vi "ATF-Storage NS Connect.vi"(8 "error in (no error)":errorcluster, 11 "Storage Ip Address":string) -> (0 "error out":errorcluster, 2 "writer endpoint":refnum<k21>, 3 "reader endpoint":refnum<k21>)   [LabVIEW 2022 SP3]
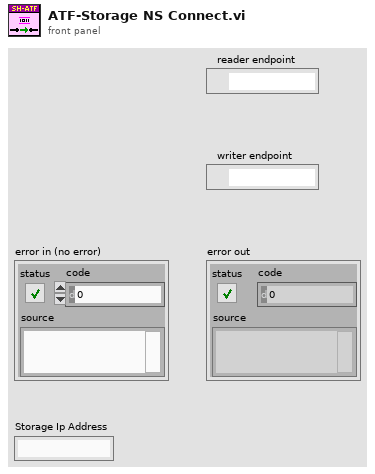
[diagram p1: front panel]
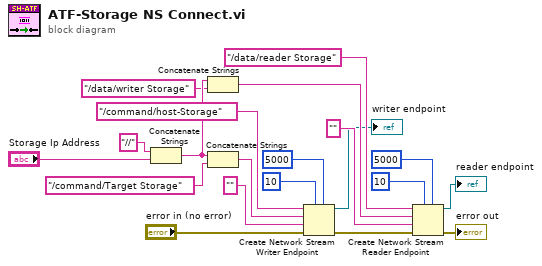
[diagram p0: block diagram]
diagram:
  n1 = Concatenate Strings("//" ("reader url"), "Storage Ip Address") -> (w16:string)
  n2 = Concatenate Strings(w16, "/data/writer Storage" ("reader url")) -> (w11:string)
  n3 = Concatenate Strings(w16, "/command/Target Storage" ("reader url")) -> (w12:string)
  n4 = Create Network Stream Writer Endpoint(5:5000 ("timeout in ms (-1)"), 7:10 ("timeout in ms (-1)"), 8:"error in (no error)", 9:"" ("concatenated string"), 10:w12, 11:"/command/host-Storage" ("writer name")) -> (0:w9:errorcluster, 3:→"writer endpoint":refnum<k21>)  [unwired: 1 in]
  n5 = Create Network Stream Reader Endpoint(5:5000 ("timeout in ms (-1)"), 7:10 ("reader buffer size"), 8:w9, 9:"" ("concatenated string"), 10:w11, 11:"/data/reader Storage" ("writer name")) -> (0:→"error out":errorcluster, 3:→"reader endpoint":refnum<k21>)  [unwired: 1 in]
